vi "main.vi"() -> ()   [LabVIEW 2015]
uses:
  Program Files/C4Utility/c4hdl/win64-x64/LabVIEW/C4Dev_writeFeature.vi
  Program Files/C4Utility/c4hdl/win64-x64/LabVIEW/C4Dev_readFeature.vi
  Program Files/C4Utility/c4hdl/win64-x64/LabVIEW/libC4HdlLV.lvlib
panel:
  out "event data out":string
  in  "event feature list":string="EventFrameStart\nEventFrameStartTimestamp\nEventFrameEnd\nEventFrameEndTimestamp"
  in  "event specific configuration":string="EventSelector = FrameStart\nEventNotification = On\nEventSelector = FrameEnd\nEventNotification = On"
  in  "camCfg in":string="# simple configuration example of heliInspect H8 using internal motion control\n#\n# Motion parameters in [mm] or [mm/s]\n# exposure ration between 0.0 and 1.0 [1.0 = 100% exposure]\n#\n# enable required components\nComponentSelector = Intensity\nComponentEnable = false\nComponentSelector = Range\nComponentEnable = true\nComponentSelector = Reflectance\nComponentEnable = true\nComponentSelector = Phase\nComponentEnable = false\n#\n# enable required chunk data (optional)\nChunkModeActive = true\nChunkSelector = PartCount\nChunkEnable = true\nChunkSelector = PartType\nChunkEnable = true\n#\n# trigger configuration\nTriggerSelector = RecordingStart\nTriggerMode = On\nTriggerSource = Stage\nTriggerSelector = AcquisitionStart\nTriggerMode = Off\nTriggerSelector = FrameStart\nTriggerMode = On\nTriggerSource = Software\n# Hint: The TriggerSource also controls the TriggerSoftware feature.\n#\n# encoder configuration\nEncoderSelector = Camera\nEncoderInverter = true\n#\n# motion and position configuration\nScanPosition = -1.4\nScanRange = 0.5\nScanSpeed = 5.0\nGeneralSpeed = 10.0\n#\nScanMode = Down\nStageInit = 1\n#\n# additional camera and processing configuration\nScan3dExtractionMethod = AcceleratedCenterOfMassIQCorrection\nScan3dScalingMethod = zTags\nScan3dDistanceUnit = um\n#\nTargetVerticalSpacing = 2.5\nExposureRatio = 1.0\n#\nFPNCorrection = AverageLastFrames\nFPNCorrectionNFrames = 8\nExtSimpMaxHWin = 7\n#\n# illumination control (D3)\nLightControllerSelector = LightController0\nLightControllerSource = UserOutput0\nLightBrightness = 100.0\n# illumination control (D2)\n# LineSelector = Line2\n# LineSource = UserOutput0\n# LineInverter = True\n# switch on the illumination (D2/D3)\nUserOutputSelector = UserOutput0\nUserOutputValue = true"
  out "acqItr":i32
  out "Surface out":dbl[][](graph)
  out "error out":errorcluster
  out "devName out":string[](array[string])
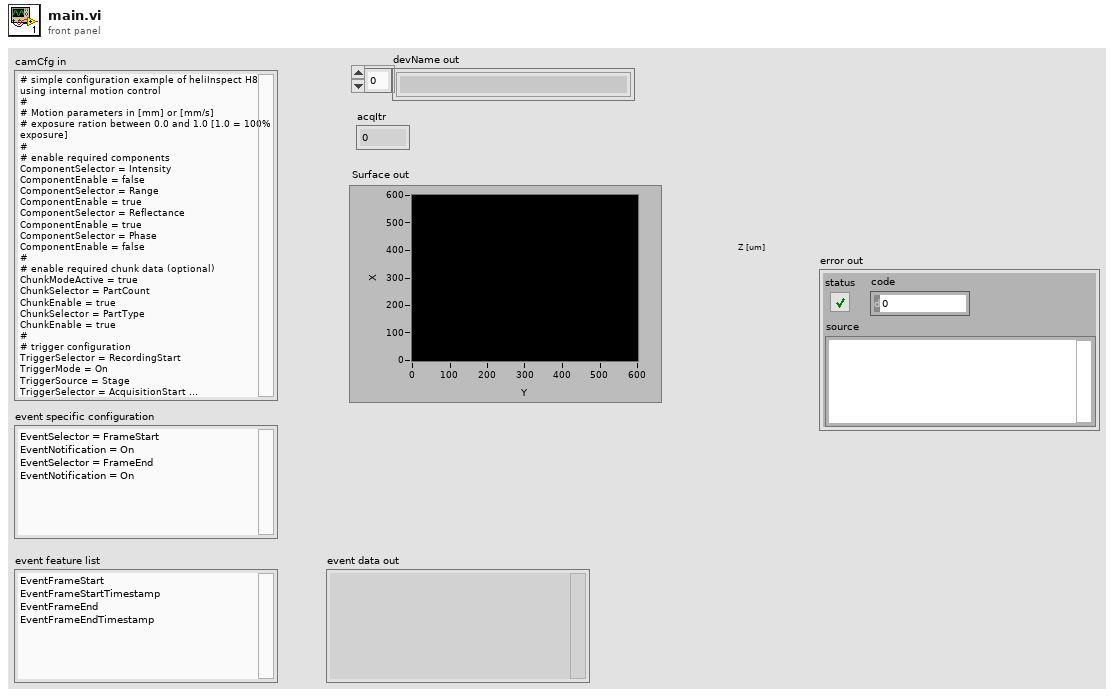
[diagram p1: front panel]
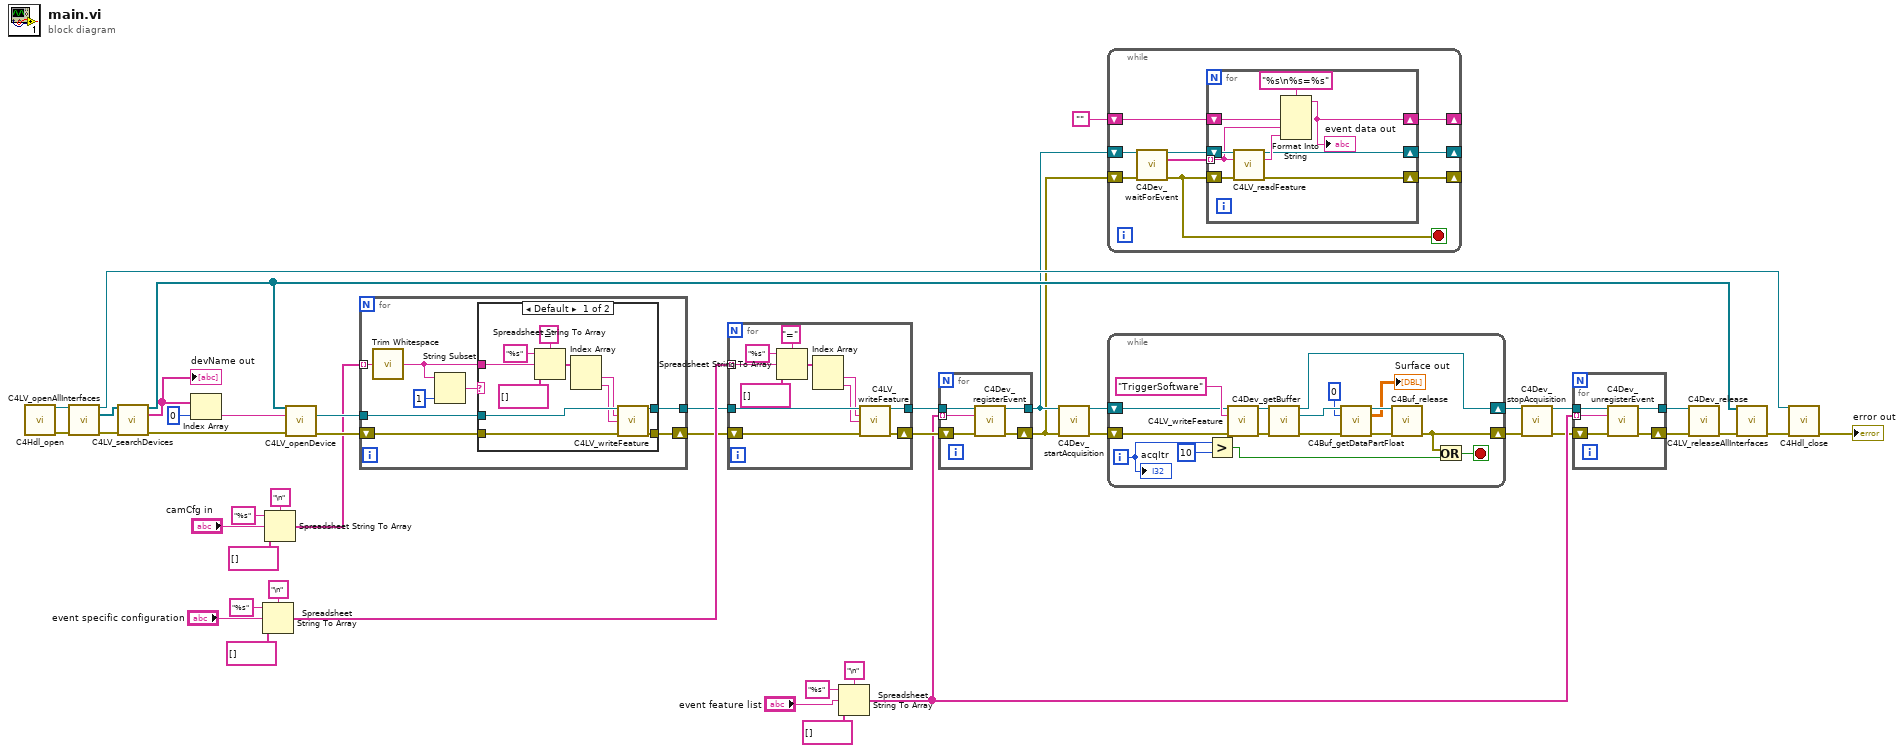
[diagram p0: block diagram]
diagram:
  n1 = call "C4Hdl_open.vi"() -> ("c4hdl out"=w43:refnum<k24>, "error out"=w44:errorcluster)  [unwired: 14 in]
  n2 = call "C4LV_openAllInterfaces.vi"("c4hdl in"=w43, "error in (no error)"=w44) -> ("c4hdl out"=w25:refnum<k24>, "c4if Arr out"=w41:refnum<k24>[], "error out"=w42:errorcluster)  [unwired: 11 in]
  n3 = call "C4LV_searchDevices.vi"("c4if Arr in"=w41, "error in (no error)"=w42) -> ("c4if Arr out"=w34:refnum<k24>[], "devName out"=w40:string[], "error out"=w39:errorcluster)  [unwired: 11 in]
  "devName out" <- w40
  n4 = Index Array(array=w40, index=0) -> (element=w38:string)
  n5 = Spreadsheet String To Array(delimiter (Tab)="\n", format string="%s", spreadsheet string="event specific configuration", array type (2D Dbl)=string[] [] ("Array Constant")) -> (array=w20:string[])
  n6 = Spreadsheet String To Array(delimiter (Tab)="\n", format string="%s", spreadsheet string="camCfg in", array type (2D Dbl)=string[] [] ("Array Constant")) -> (array=w1:string[])
  n7 = call "C4LV_openDevice.vi"("c4if Arr in"=w34, "devName in"=w38, "error in (no error)"=w39) -> ("c4dev out"=w2:refnum<k24>, "error out"=w5:errorcluster)  [unwired: 10 in, 1 out]
  n8 = for {
    tunnel: w1 -> [w49] mode=indexing
    tunnel: w2 -> [w50]
    shift-right: [w52] -> w4
    shift-left: w5 -> [w53]
    tunnel: [w51] -> w3
    n9 = call <vilib>:"Trim Whitespace.vi"("string"=w49) -> ("trimmed string"=w48:string)  [unwired: 1 in]
    n10 = String Subset(string=w48, length (rest)=1 ("length (rest)")) -> (substring=w47:string)  [unwired: 1 in]
    n11 = case shown="Default" w47 {
      tunnel: w53 -> [w64 w66]
      tunnel: [w63 w66] -> w52
      tunnel: [w62 w65] -> w51
      tunnel: w50 -> [w61 w65]
      tunnel: w48 -> [w56 _]
      frame Default {
        n12 = Spreadsheet String To Array(delimiter (Tab)="=", format string="%s", spreadsheet string=w56, array type (2D Dbl)=string[] [] ("Array Constant")) -> (array=w60:string[])
        n13 = Index Array(array=w60) -> (element #1=w54:string, element #2=w55:string)  [unwired: 2 in]
        n14 = call-poly "C4LV_writeFeature.vi"("c4dev in"=w61, "name in"=w54, "value in"=w55, "error in"=w64) -> ("c4dev out"=w62:refnum<k24>, "error out"=w63:errorcluster)  [unwired: 10 in]
      }
      frame "#" {
        # "# is a comment"
      }
    }
  }
  n15 = for {
    tunnel: w20 -> [w69] mode=indexing
    tunnel: w3 -> [w74]
    shift-right: [w76] -> w15
    shift-left: w4 -> [w77]
    tunnel: [w75] -> w14
    n16 = Spreadsheet String To Array(delimiter (Tab)="=", format string="%s", spreadsheet string=w69, array type (2D Dbl)=string[] [] ("Array Constant")) -> (array=w73:string[])
    n17 = Index Array(array=w73) -> (element #1=w67:string, element #2=w68:string)  [unwired: 2 in]
    n18 = call-poly "C4LV_writeFeature.vi"("c4dev in"=w74, "name in"=w67, "value in"=w68, "error in"=w77) -> ("c4dev out"=w75:refnum<k24>, "error out"=w76:errorcluster)  [unwired: 10 in]
  }
  n19 = Spreadsheet String To Array(delimiter (Tab)="\n", format string="%s", spreadsheet string="event feature list", array type (2D Dbl)=string[] [] ("Array Constant")) -> (array=w13:string[])
  n20 = for {
    tunnel: w13 -> [w82] mode=indexing
    shift-right: [w80] -> w7
    shift-left: w15 -> [w81]
    tunnel: w14 -> [w79]
    tunnel: [w78] -> w8
    n21 = call "C4Dev_registerEvent.vi"("c4dev in"=w79, "name in"=w82, "error in"=w81) -> ("c4dev out"=w78:refnum<k24>, "error out"=w80:errorcluster)  [unwired: 11 in]
  }
  n22 = call "C4Dev_startAcquisition.vi"("c4dev in"=w8, "error in (no error)"=w7) -> ("c4dev out"=w37:refnum<k24>, "error out"=w36:errorcluster)  [unwired: 12 in]
  n23 = while {
    shift-right: [w84] -> _
    shift-left: w7 -> [w90]
    shift-right: [w85] -> _
    shift-left: "" -> [w86]
    shift-right: [w83] -> _
    shift-left: w8 -> [w91]
    stop <- w87 stop-if-true
    n24 = call "C4Dev_waitForEvent.vi"("c4dev in"=w91, "error in"=w90) -> ("c4dev out"=w88:refnum<k24>, "feature names out"=w89:string[], "error out"=w87:errorcluster)  [unwired: 11 in]
    n25 = for {
      tunnel: w89 -> [w96] mode=indexing
      shift-right: [w92] -> w85
      shift-left: w86 -> [w97]
      shift-right: [w93] -> w84
      shift-left: w87 -> [w100]
      shift-right: [w94] -> w83
      shift-left: w88 -> [w99]
      n26 = call-poly "C4LV_readFeature.vi"("c4dev in"=w99, "name in"=w96, "error in"=w100) -> ("c4dev out"=w94:refnum<k24>, "value out"=w95:string, "error out"=w93:errorcluster)  [unwired: 10 in]
      n27 = Format Into String(format string="%s\n%s=%s" ("delimiter (Tab)"), w97, w96, w95) -> (resulting string=w92:string)  [unwired: 2 in, 1 out]
      "event data out" <- w92
    }
  }
  n28 = while {
    shift-right: [w106] -> w33
    shift-left: w36 -> [w107]
    shift-right: [w101] -> w32
    shift-left: w37 -> [w104]
    i -> [w117]
    stop <- w114 stop-if-true
    n29 = Greater?(x=w117, y=10) -> (0:w115:bool)
    n30 = call-poly "C4LV_writeFeature.vi"("c4dev in"=w104, "name in"="TriggerSoftware", "error in"=w107) -> ("c4dev out"=w113:refnum<k24>, "error out"=w108:errorcluster)  [unwired: 11 in]
    n31 = call "C4Dev_getBuffer.vi"("c4dev in"=w113, "error in (no error)"=w108) -> ("c4dev out"=w101:refnum<k24>, "c4buf out"=w111:refnum<k24>, "error out"=w109:errorcluster)  [unwired: 11 in]
    n32 = call "C4Buf_getDataPartFloat.vi"("c4buf in"=w111, "partIdx in"=i64 0, "error in (no error)"=w109) -> ("c4buf out"=w112:refnum<k24>, "data out"=→"Surface out":dbl[][], "error out"=w110:errorcluster)  [unwired: 10 in]
    n33 = call "C4Buf_release.vi"("c4buf in"=w112, "error in (no error)"=w110) -> ("error out"=w106:errorcluster)  [unwired: 13 in]
    n34 = Or(x=w106, y=w115) -> (x .or. y?=w114:bool)
    "acqItr" <- w117
  }
  n35 = call "C4Dev_stopAcquisition.vi"("c4dev in"=w32, "error in (no error)"=w33) -> ("c4dev out"=w12:refnum<k24>, "error out"=w9:errorcluster)  [unwired: 12 in]
  n36 = for {
    tunnel: w13 -> [w120] mode=indexing
    shift-right: [w121] -> w10
    shift-left: w9 -> [w122]
    tunnel: w12 -> [w119]
    tunnel: [w118] -> w11
    n37 = call "C4Dev_unregisterEvent.vi"("c4dev in"=w119, "name in"=w120, "error in"=w122) -> ("c4dev out"=w118:refnum<k24>, "error out"=w121:errorcluster)  [unwired: 11 in]
  }
  n38 = call "C4Dev_release.vi"("c4dev in"=w11, "error in (no error)"=w10) -> ("error out"=w35:errorcluster)  [unwired: 13 in]
  n39 = call "C4LV_releaseAllInterfaces.vi"("c4if Arr in"=w34, "error in (no error)"=w35) -> ("error out"=w27:errorcluster)  [unwired: 13 in]
  n40 = call "C4Hdl_close.vi"("c4hdl in"=w25, "error in (no error)"=w27) -> ("error out"=→"error out":errorcluster)  [unwired: 13 in]
